vi "Initialize.vi"(8 "error in (no error)":errorcluster, 11 "S4ACS_GUI in":refnum<class "S4GUI.lvclass">) -> (0 "error out":errorcluster, 3 "S4ACS_GUI out":refnum<class "S4GUI.lvclass">)   [LabVIEW 2018, in "S4GUI.lvclass"]
uses:
  S4GUI.lvclass
  S4GUI.lvclass/S4GUI.ctl
  Publisher/Publisher.lvclass
  GSserver/GSserver.lvclass
  WeatherStation/WeatherStation.lvclass
  TelFocus/TelFocus.lvclass
  TCS/TCS.lvclass
  Instrument/Instrument.lvclass
  Acquisition/Acquisition.lvclass
  SyncBox/Sync Box.lvclass
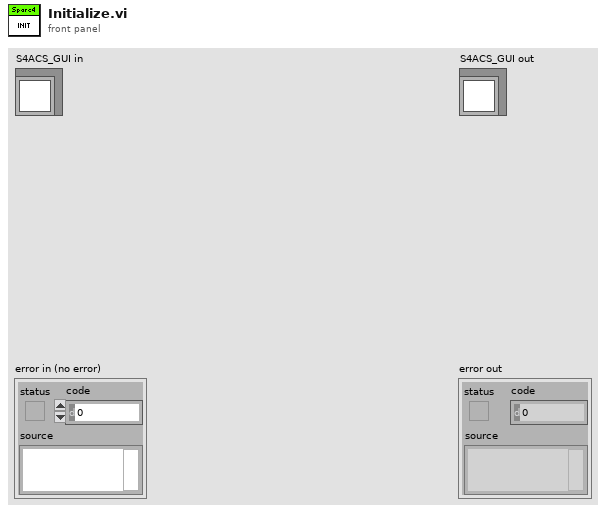
[diagram p1: front panel]
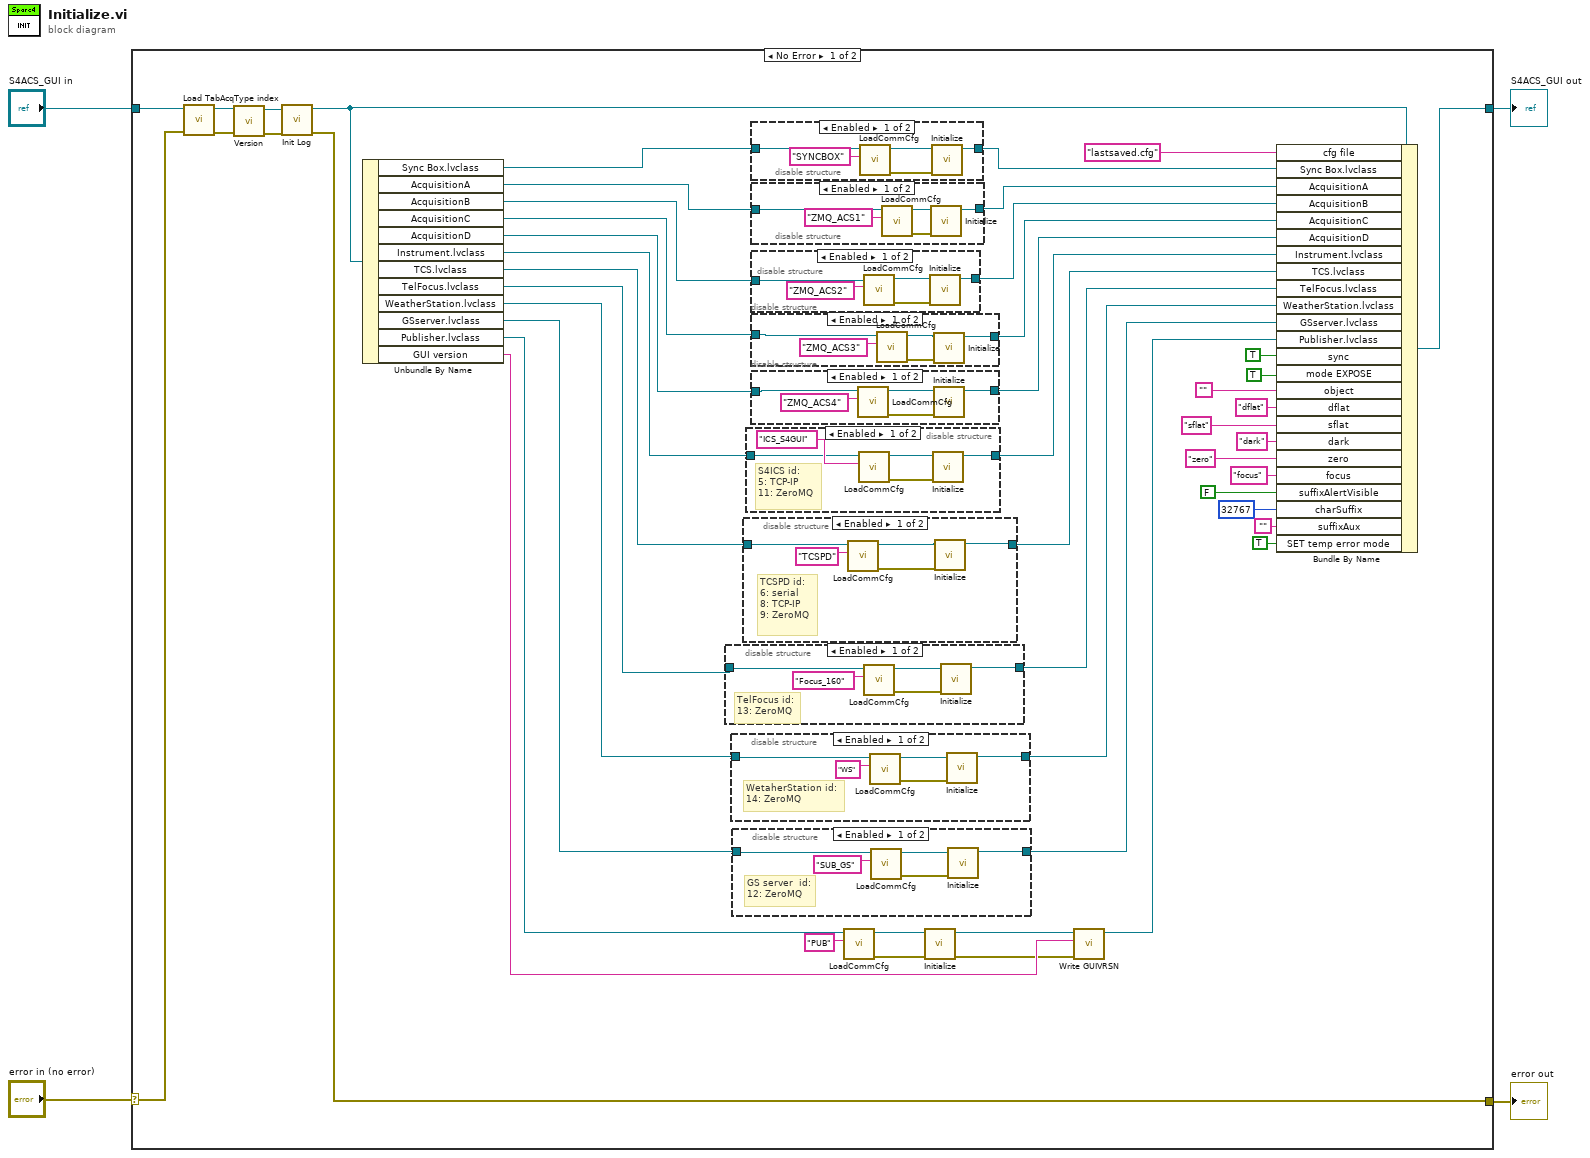
[diagram p0: block diagram]
diagram:
  n1 = case shown="No Error" "error in (no error)" {
    selector: "error in (no error)" -> [w18 w116]
    tunnel: [w21 w116] -> w3
    tunnel: [w33 w115] -> w1
    tunnel: "S4ACS_GUI in" -> [w16 w115]
    frame No Error {
      n2 = call-dynamic "Load TabAcqType index.vi"("error in (no error)"=w18, "S4GUI in"=w16) -> ("error out"=w17:errorcluster, "S4GUI out"=w15:refnum<class "S4GUI.lvclass">)  [unwired: 8 in]
      n3 = call-dynamic "Version.vi"("error in (no error)"=w17, "S4GUI in"=w15) -> ("error out"=w20:errorcluster, "S4GUI out"=w19:refnum<class "S4GUI.lvclass">)  [unwired: 8 in]
      n4 = call-dynamic "Init Log.vi"("error in (no error)"=w20, "S4GUI in"=w19) -> ("error out"=w21:errorcluster, "S4GUI out"=w39:refnum<class "S4GUI.lvclass">)  [unwired: 8 in]
      n5 = Unbundle By Name(w39) -> ("Sync Box.lvclass"=w45:refnum<class "Sync Box.lvclass">, "AcquisitionA"=w52:refnum<class "Acquisition.lvclass">, "AcquisitionB"=w51:refnum<class "Acquisition.lvclass">, "AcquisitionC"=w50:refnum<class "Acquisition.lvclass">, "AcquisitionD"=w49:refnum<class "Acquisition.lvclass">, "Instrument.lvclass"=w44:refnum<class "Instrument.lvclass">, "TCS.lvclass"=w41:refnum<class "TCS.lvclass">, "TelFocus.lvclass"=w38:refnum<class "TelFocus.lvclass">, "WeatherStation.lvclass"=w36:refnum<class "WeatherStation.lvclass">, "GSserver.lvclass"=w23:refnum<class "GSserver.lvclass">, "Publisher.lvclass"=w32:refnum<class "Publisher.lvclass">, "GUI version"=w27:string)
      n6 = disable-structure shown="Enabled" {
        disable-tunnel: w38 -> [w68 w72]
        disable-tunnel: [w67 w72] -> w37
        frame Enabled {
          # "TelFocus id:\n13: ZeroMQ"
          n7 = call-dynamic "LoadCommCfg.vi"("section (server name)"="Focus_160", "Server in"=w68) -> ("error out"=w69:errorcluster, "Server out"=w70:refnum<class "TelFocus.lvclass">)  [unwired: 8 in]
          n8 = call-dynamic "Initialize.vi"("error in (no error)"=w69, "TelFocus in"=w70) -> ("TelFocus out"=w67:refnum<class "TelFocus.lvclass">)  [unwired: 8 in, 1 out]
        }
        frame Disabled {
        }
      }
      n9 = disable-structure shown="Enabled" {
        disable-tunnel: w36 -> [w62 w66]
        disable-tunnel: [w61 w66] -> w34
        frame Enabled {
          # "WetaherStation id:\n14: ZeroMQ"
          n10 = call-dynamic "LoadCommCfg.vi"("section (server name)"="WS", "Server in"=w62) -> ("error out"=w63:errorcluster, "Server out"=w64:refnum<class "WeatherStation.lvclass">)  [unwired: 8 in]
          n11 = call-dynamic "Initialize.vi"("error in (no error)"=w63, "WeatherStation in"=w64) -> ("WeatherStation out"=w61:refnum<class "WeatherStation.lvclass">)  [unwired: 8 in, 1 out]
        }
        frame Disabled {
        }
      }
      n12 = disable-structure shown="Enabled" {
        disable-tunnel: w23 -> [w56 w60]
        disable-tunnel: [w55 w60] -> w22
        frame Enabled {
          # "GS server  id:\n12: ZeroMQ"
          n13 = call-dynamic "LoadCommCfg.vi"("section (server name)"="SUB_GS", "Server in"=w56) -> ("error out"=w57:errorcluster, "Server out"=w58:refnum<class "GSserver.lvclass">)  [unwired: 8 in]
          n14 = call-dynamic "Initialize.vi"("error in (no error)"=w57, "GSserver in"=w58) -> ("GSserver out"=w55:refnum<class "GSserver.lvclass">)  [unwired: 8 in, 1 out]
        }
        frame Disabled {
        }
      }
      n15 = disable-structure shown="Enabled" {
        disable-tunnel: w41 -> [w93 w96]
        disable-tunnel: [w95 w96] -> w40
        frame Enabled {
          # "TCSPD id:\n6: serial \n8: TCP-IP\n9: ZeroMQ"
          n16 = call-dynamic "LoadCommCfg.vi"("section (server name)"="TCSPD", "Server in"=w93) -> ("error out"=w91:errorcluster, "Server out"=w92:refnum<class "TCS.lvclass">)  [unwired: 8 in]
          n17 = call-dynamic "Initialize.vi"("error in (no error)"=w91, "TCS in"=w92) -> ("TCS out"=w95:refnum<class "TCS.lvclass">)  [unwired: 8 in, 1 out]
        }
        frame Disabled {
        }
      }
      n18 = disable-structure shown="Enabled" {
        disable-tunnel: w44 -> [w87 w90]
        disable-tunnel: [w89 w90] -> w43
        frame Enabled {
          # "S4ICS id:\n5: TCP-IP\n11: ZeroMQ"
          n19 = call-dynamic "LoadCommCfg.vi"("section (server name)"="ICS_S4GUI", "Server in"=w87) -> ("error out"=w85:errorcluster, "Server out"=w86:refnum<class "Instrument.lvclass">)  [unwired: 8 in]
          n20 = call-dynamic "Initialize.vi"("error in (no error)"=w85, "Instrument in"=w86) -> ("Instrument out"=w89:refnum<class "Instrument.lvclass">)  [unwired: 8 in, 1 out]
        }
        frame Disabled {
        }
      }
      n21 = disable-structure shown="Enabled" {
        disable-tunnel: [w113 w114] -> w46
        disable-tunnel: w45 -> [w112 w114]
        frame Enabled {
          n22 = call-dynamic "LoadCommCfg.vi"("section (server name)"="SYNCBOX", "Server in"=w112) -> ("error out"=w110:errorcluster, "Server out"=w111:refnum<class "Sync Box.lvclass">)  [unwired: 8 in]
          n23 = call-dynamic "Initialize.vi"("error in (no error)"=w110, "Sync Box in"=w111) -> ("Sync Box out"=w113:refnum<class "Sync Box.lvclass">)  [unwired: 8 in, 1 out]
        }
        frame Disabled {
        }
      }
      n24 = disable-structure shown="Enabled" {
        disable-tunnel: [w107 w108] -> w54
        disable-tunnel: w52 -> [w106 w108]
        frame Enabled {
          n25 = call-dynamic "LoadCommCfg.vi"("section (server name)"="ZMQ_ACS1", "Server in"=w106) -> ("error out"=w104:errorcluster, "Server out"=w105:refnum<class "Acquisition.lvclass">)  [unwired: 8 in]
          n26 = call-dynamic "Initialize.vi"("error in (no error)"=w104, "Acquisition in"=w105) -> ("Acquisition out"=w107:refnum<class "Acquisition.lvclass">)  [unwired: 8 in, 1 out]
        }
        frame Disabled {
        }
      }
      n27 = disable-structure shown="Enabled" {
        disable-tunnel: [w101 w102] -> w53
        disable-tunnel: w51 -> [w99 w102]
        frame Enabled {
          n28 = call-dynamic "LoadCommCfg.vi"("section (server name)"="ZMQ_ACS2", "Server in"=w99) -> ("error out"=w97:errorcluster, "Server out"=w98:refnum<class "Acquisition.lvclass">)  [unwired: 8 in]
          n29 = call-dynamic "Initialize.vi"("error in (no error)"=w97, "Acquisition in"=w98) -> ("Acquisition out"=w101:refnum<class "Acquisition.lvclass">)  [unwired: 8 in, 1 out]
        }
        frame Disabled {
        }
      }
      n30 = disable-structure shown="Enabled" {
        disable-tunnel: w50 -> [w81 w84]
        disable-tunnel: [w83 w84] -> w48
        frame Enabled {
          n31 = call-dynamic "LoadCommCfg.vi"("section (server name)"="ZMQ_ACS3", "Server in"=w81) -> ("error out"=w79:errorcluster, "Server out"=w80:refnum<class "Acquisition.lvclass">)  [unwired: 8 in]
          n32 = call-dynamic "Initialize.vi"("error in (no error)"=w79, "Acquisition in"=w80) -> ("Acquisition out"=w83:refnum<class "Acquisition.lvclass">)  [unwired: 8 in, 1 out]
        }
        frame Disabled {
        }
      }
      n33 = disable-structure shown="Enabled" {
        disable-tunnel: w49 -> [w75 w78]
        disable-tunnel: [w77 w78] -> w47
        frame Enabled {
          n34 = call-dynamic "LoadCommCfg.vi"("section (server name)"="ZMQ_ACS4", "Server in"=w75) -> ("error out"=w73:errorcluster, "Server out"=w74:refnum<class "Acquisition.lvclass">)  [unwired: 8 in]
          n35 = call-dynamic "Initialize.vi"("error in (no error)"=w73, "Acquisition in"=w74) -> ("Acquisition out"=w77:refnum<class "Acquisition.lvclass">)  [unwired: 8 in, 1 out]
        }
        frame Disabled {
        }
      }
      n36 = call-dynamic "LoadCommCfg.vi"("section (server name)"="PUB", "Client in"=w32) -> ("error out"=w30:errorcluster, "Client out"=w31:refnum<class "Publisher.lvclass">)  [unwired: 8 in]
      n37 = call-dynamic "Initialize.vi"("error in (no error)"=w30, "Client in"=w31) -> ("error out"=w26:errorcluster, "Client out"=w28:refnum<class "Publisher.lvclass">)  [unwired: 8 in]
      n38 = call-dynamic "Write GUIVRSN.vi"("error in (no error)"=w26, "GUIVRSN"=w27, "Publisher in"=w28) -> ("Publisher out"=w24:refnum<class "Publisher.lvclass">)  [unwired: 7 in, 1 out]
      n39 = Bundle By Name(cluster=w39, "cfg file"="lastsaved.cfg", "Sync Box.lvclass"=w46, "AcquisitionA"=w54, "AcquisitionB"=w53, "AcquisitionC"=w48, "AcquisitionD"=w47, "Instrument.lvclass"=w43, "TCS.lvclass"=w40, "TelFocus.lvclass"=w37, "WeatherStation.lvclass"=w34, "GSserver.lvclass"=w22, "Publisher.lvclass"=w24, "sync"=TRUE, "mode EXPOSE"=TRUE, "object"="" ("ClusterSuffix.object"), "dflat"="dflat" ("ClusterSuffix.dflat"), "sflat"="sflat" ("ClusterSuffix.sflat"), "dark"="dark" ("ClusterSuffix.dark"), "zero"="zero" ("ClusterSuffix.zero"), "focus"="focus" ("ClusterSuffix.focus"), "suffixAlertVisible"=FALSE, "charSuffix"=i16 32767 ("charKeyboard"), "suffixAux"="", "SET temp error mode"=TRUE) -> (w33:refnum<class "S4GUI.lvclass">)
    }
    frame Error {
    }
  }
  "error out" <- w3
  "S4ACS_GUI out" <- w1
